vi "Get XML Object tag.vi"(8 "error in (no error)":errorcluster, 11 "Refnum in":refnum<k20>) -> (0 "error out":errorcluster, 2 "FirstChild":refnum<k20>, 3 "Refnum out":refnum<k20>)   [LabVIEW 2018, in "Serializer.lvclass"]
uses:
  Serializer.lvclass
  <resource>/objmgr/DOMUserDefRef.rc
panel:
  out "XML 6":string
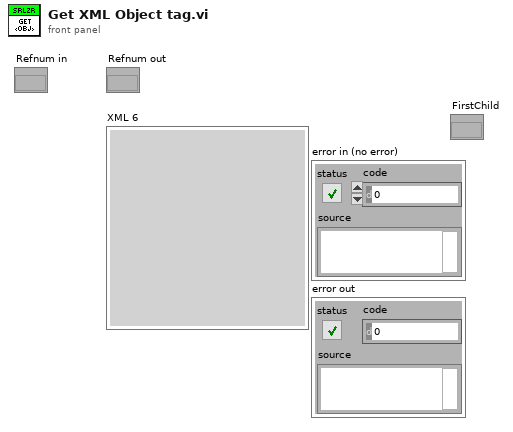
[diagram p1: front panel]
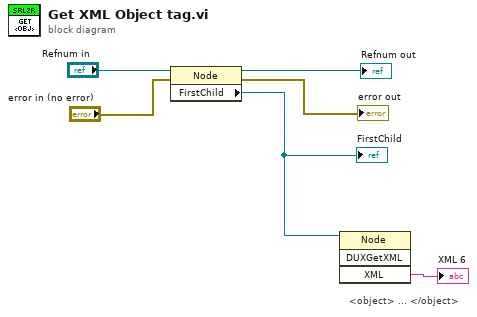
[diagram p0: block diagram]
diagram:
  # "<object> ... </object>"
  n1 = property class="Node"(reference="Refnum in", error in="error in (no error)") -> (error out=→"error out":errorcluster, "FirstChild"=w3:refnum<k20>)  [unwired: 1 out]
  "FirstChild" <- w3
  n2 = invoke class="Node" method="DUXGetXML"(reference=w3) -> ("XML"=→"XML 6":string)  [unwired: 3 in, 3 out]
  "Refnum out" <- "Refnum in"
